vi "LDA_header.vi"() -> (0 "LDA Header string":string)   [LabVIEW 2010]
uses:
  Globals/Meas_global.vi
  Globals/LDA_meas_global_1.vi
  Globals/LDA_meas_global_2.vi
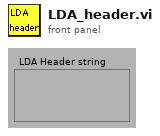
[diagram p1: front panel]
types:
  T1 = typedef "BSA_info_Cluster.ctl" = cluster{"GPIB Address":string, "No of Check Bytes":i32, "Extra Info":string, "COLOUR":u32, "Wavelength (nm)":dbl}
  T2 = cluster{"Arrival time clock":enum16{"External", "Internal"}, "Clock source":enum16{"Slave", "Master", "Private"}, "Coincidence":enum16{"Slave", "Master", "Private"}}
  T3 = cluster{"Dead time (s)":dbl, "Duty cycle (%)":dbl, "Data collection mode":enum16{"Burst", "Contiuous", "Dead time", "External"}}
  T4 = enum16{"Burst", "Contiuous", "Dead time", "External"}
  T5 = cluster{"Burst criterion":enum16{"Envelope", "Pedestal", "Env and ped"}, "Oversize reject level":enum16{"1 (disabled)", "2", "3", "4", "5", "6", "7", "8", "9"}, "Pedestal attenuation":enum16{"0", "6", "12", "18"}, "Record length":enum16{"8", "16", "32", "64"}, "Quality factor":i16}
  T6 = enum16{"1 (disabled)", "2", "3", "4", "5", "6", "7", "8", "9"}
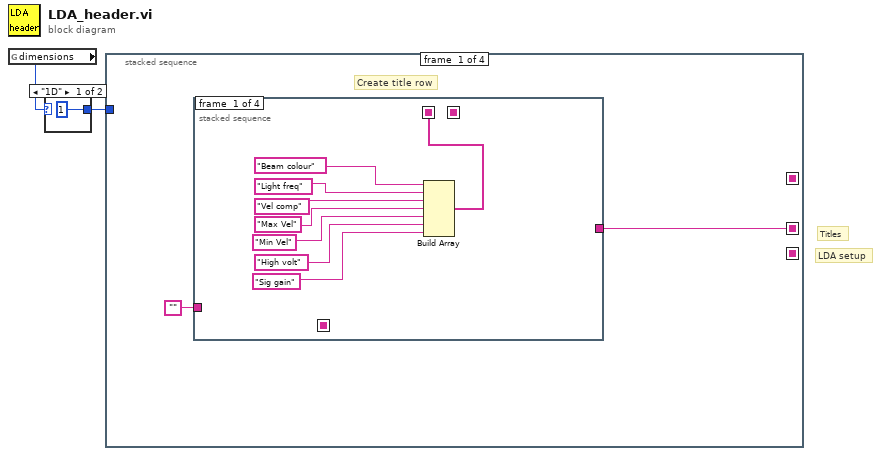
[diagram p0: block diagram]
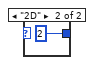
[diagram p2: hidden frame]
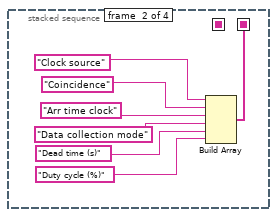
[diagram p3: hidden frame]
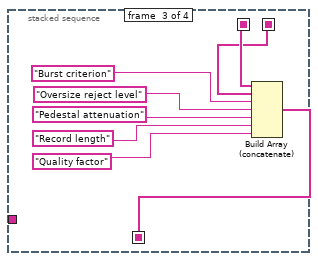
[diagram p4: hidden frame]
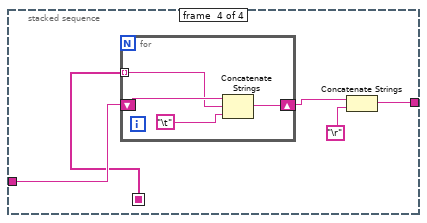
[diagram p5: hidden frame]
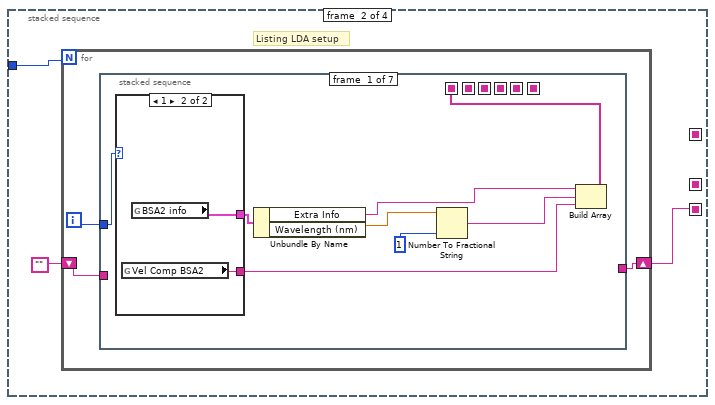
[diagram p6: hidden frame]
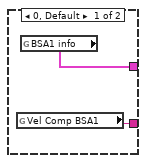
[diagram p7: hidden frame]
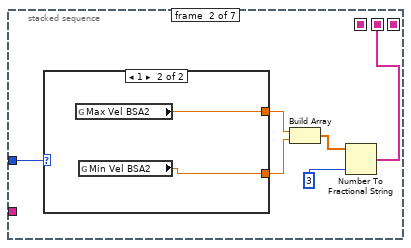
[diagram p8: hidden frame]
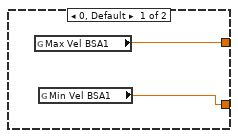
[diagram p9: hidden frame]
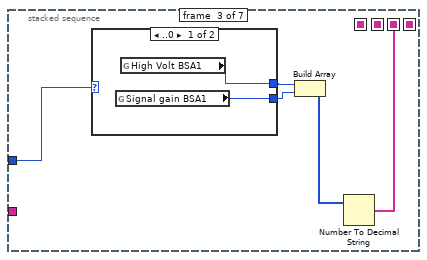
[diagram p10: hidden frame]
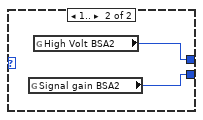
[diagram p11: hidden frame]
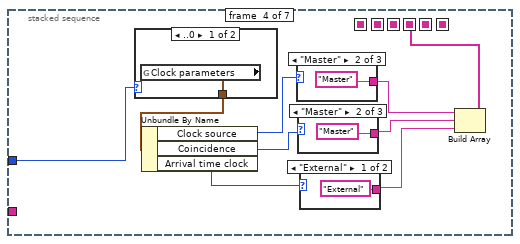
[diagram p12: hidden frame]
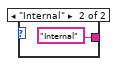
[diagram p13: hidden frame]
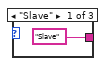
[diagram p14: hidden frame]
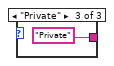
[diagram p15: hidden frame]
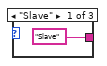
[diagram p16: hidden frame]
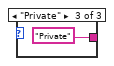
[diagram p17: hidden frame]
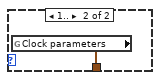
[diagram p18: hidden frame]
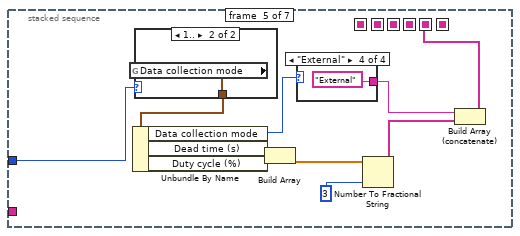
[diagram p19: hidden frame]
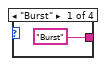
[diagram p20: hidden frame]
diagram:
  # "LDA setup"
  # "Titles"
  n1 = global read "Meas_global.vi" "dimensions"() -> (w2:enum16{"1D", "2D"})
  n2 = case shown="\"1D\"" w2 {
    tunnel: [1 2] -> w1
    frame "1D" {
    }
    frame "2D" {
    }
  }
  n3 = stacked-sequence {
    seq-local: [w6 _ _ _] -> [_ _ _ w174]
    seq-local: [_ w41 _ _] -> [_ _ _ w173]
    seq-local: [_ _ w164 _] -> [_ _ _ w176]
    tunnel: w1 -> [_ w39 _ _]
    frame #0 {
      # "Create title row"
      n4 = stacked-sequence {
        seq-local: [w7 _ _ _] -> [_ _ w24 _]
        seq-local: [_ w15 _ _] -> [_ _ w23 _]
        seq-local: [_ _ w22 _] -> [_ _ _ w33]
        tunnel: "" -> [_ _ _ w34]
        tunnel: [_ _ _ w31] -> w6
        frame #0 {
          n5 = Build Array("Beam colour", "Light freq", "Vel comp", "Max Vel", "Min Vel", "High volt", "Sig gain") -> (w7:string[])
        }
        frame #1 {
          n6 = Build Array("Clock source", "Coincidence", "Arr time clock", "Data collection mode", "Dead time (s)", "Duty cycle (%)") -> (w15:string[])
        }
        frame #2 {
          n7 = Build Array (concatenate)(w24, w23, "Burst criterion", "Oversize reject level", "Pedestal attenuation", "Record length", "Quality factor") -> (w22:string[])
        }
        frame #3 {
          n8 = for {
            shift-right: [w37] -> w32
            shift-left: w34 -> [w38]
            tunnel: w33 -> [w35] mode=indexing
            n9 = Concatenate Strings(w38, w35, "\t") -> (w37:string)
          }
          n10 = Concatenate Strings(w32, "\r") -> (w31:string)
        }
      }
    }
    frame #1 {
      # "Listing LDA setup"
      n11 = for {
        N: w39 -> [_]
        shift-right: [w42] -> w41
        shift-left: "" -> [w43]
        i -> [w44]
        n12 = stacked-sequence {
          seq-local: [_ w61 _ _ _ _ _] -> [_ _ _ _ _ _ w155]
          seq-local: [w48 _ _ _ _ _ _] -> [_ _ _ _ _ _ w156]
          seq-local: [_ _ w69 _ _ _ _] -> [_ _ _ _ _ _ w154]
          seq-local: [_ _ _ w76 _ _ _] -> [_ _ _ _ _ _ w153]
          seq-local: [_ _ _ _ w95 _ _] -> [_ _ _ _ _ _ w152]
          seq-local: [_ _ _ _ _ w111 _] -> [_ _ _ _ _ _ w151]
          tunnel: w44 -> [w52 w57 w71 w84 w104 w123 _]
          tunnel: w43 -> [_ _ _ _ _ _ w149]
          tunnel: [_ _ _ _ _ _ w148] -> w42
          frame #0 {
            n13 = case shown="1" w52 {
              tunnel: [w54 w56] -> w47
              tunnel: [w53 w55] -> w46
              frame 0, Default {
                n14 = global read "LDA_meas_global_1.vi" "Vel Comp BSA1"() -> (w53:string)
                n15 = global read "LDA_meas_global_1.vi" "BSA1 info"() -> (w54:T1)
              }
              frame 1 {
                n16 = global read "LDA_meas_global_2.vi" "Vel Comp BSA2"() -> (w55:string)
                n17 = global read "LDA_meas_global_2.vi" "BSA2 info"() -> (w56:T1)
              }
            }
            n18 = Unbundle By Name(w47) -> ("Extra Info"=w45:string, "Wavelength (nm)"=w50:dbl)
            n19 = Number To Fractional String(number=w50, precision (6)=1) -> (F-format string=w49:string)  [unwired: 2 out]
            n20 = Build Array(w45, w49, w46) -> (w48:string[])
          }
          frame #1 {
            n21 = case shown="1" w57 {
              tunnel: [w64 w66] -> w60
              tunnel: [w63 w65] -> w59
              frame 0, Default {
                n22 = global read "LDA_meas_global_1.vi" "Max Vel BSA1"() -> (w64:dbl)
                n23 = global read "LDA_meas_global_1.vi" "Min Vel BSA1"() -> (w63:dbl)
              }
              frame 1 {
                n24 = global read "LDA_meas_global_2.vi" "Max Vel BSA2"() -> (w66:dbl)
                n25 = global read "LDA_meas_global_2.vi" "Min Vel BSA2"() -> (w65:dbl)
              }
            }
            n26 = Build Array(w60, w59) -> (w58:dbl[])
            n27 = Number To Fractional String(number=w58, precision (6)=3) -> (F-format string=w61:string[])  [unwired: 2 out]
          }
          frame #2 {
            n28 = case shown="..0" w71 {
              tunnel: [w73 w75] -> w68
              tunnel: [w72 w74] -> w67
              frame ..0 {
                n29 = global read "LDA_meas_global_1.vi" "Signal gain BSA1"() -> (w72:i16)
                n30 = global read "LDA_meas_global_1.vi" "High Volt BSA1"() -> (w73:i16)
              }
              frame 1.. {
                n31 = global read "LDA_meas_global_2.vi" "Signal gain BSA2"() -> (w74:i16)
                n32 = global read "LDA_meas_global_2.vi" "High Volt BSA2"() -> (w75:i16)
              }
            }
            n33 = Build Array(w68, w67) -> (w70:i16[])
            n34 = Number To Decimal String(number=w70) -> (decimal integer string=w69:string[])  [unwired: 1 out]
          }
          frame #3 {
            n35 = case shown="..0" w84 {
              tunnel: [w93 w94] -> w83
              frame ..0 {
                n36 = global read "LDA_meas_global_1.vi" "Clock parameters"() -> (w93:T2)
              }
              frame 1.. {
                n37 = global read "LDA_meas_global_2.vi" "Clock parameters"() -> (w94:T2)
              }
            }
            n38 = Unbundle By Name(w83) -> ("Clock source"=w81:enum16{"Slave", "Master", "Private"}, "Coincidence"=w82:enum16{"Slave", "Master", "Private"}, "Arrival time clock"=w78:enum16{"External", "Internal"})
            n39 = case shown="\"Master\"" w81 {
              tunnel: ["Slave" "Master" "Private"] -> w80
              frame "Slave" {
              }
              frame "Master" {
              }
              frame "Private" {
              }
            }
            n40 = case shown="\"Master\"" w82 {
              tunnel: ["Slave" "Master" "Private"] -> w79
              frame "Slave" {
              }
              frame "Master" {
              }
              frame "Private" {
              }
            }
            n41 = case shown="\"External\"" w78 {
              tunnel: ["External" "Internal"] -> w77
              frame "External" {
              }
              frame "Internal" {
              }
            }
            n42 = Build Array(w80, w79, w77) -> (w76:string[])
          }
          frame #4 {
            n43 = case shown="1.." w104 {
              tunnel: [w109 w110] -> w103
              frame ..0 {
                n44 = global read "LDA_meas_global_1.vi" "Data collection mode"() -> (w109:T3)
              }
              frame 1.. {
                n45 = global read "LDA_meas_global_2.vi" "Data collection mode"() -> (w110:T3)
              }
            }
            n46 = Unbundle By Name(w103) -> ("Data collection mode"=w102:T4, "Dead time (s)"=w98:dbl, "Duty cycle (%)"=w97:dbl)
            n47 = Build Array(w98, w97) -> (w99:dbl[])
            n48 = case shown="\"External\"" w102 {
              tunnel: ["Burst" "Continuous" "Dead time" "External"] -> w101
              frame "Burst" {
              }
              frame "Contiuous" {
              }
              frame "Dead time" {
              }
              frame "External" {
              }
            }
            n49 = Number To Fractional String(number=w99, precision (6)=3) -> (F-format string=w96:string[])  [unwired: 2 out]
            n50 = Build Array (concatenate)(w101, w96) -> (w95:string[])
          }
          frame #5 {
            n51 = case shown="1.." w123 {
              tunnel: [w144 w145] -> w122
              frame ..0 {
                n52 = global read "LDA_meas_global_1.vi" "Analysis parameters"() -> (w144:T5)
              }
              frame 1.. {
                n53 = global read "LDA_meas_global_2.vi" "Analysis parameters"() -> (w145:T5)
              }
            }
            n54 = Unbundle By Name(w122) -> ("Burst criterion"=w120:enum16{"Envelope", "Pedestal", "Env and ped"}, "Oversize reject level"=w121:T6, "Pedestal attenuation"=w117:enum16{"0", "6", "12", "18"}, "Record length"=w115:enum16{"8", "16", "32", "64"}, "Quality factor"=w114:i16)
            n55 = case shown="\"Envelope\"" w120 {
              tunnel: ["Envelope" "Pedestal" "Env and ped"] -> w119
              frame "Envelope" {
              }
              frame "Pedestal" {
              }
              frame "Env and ped" {
              }
            }
            n56 = case shown="\"1 (disabled)\"" w121 {
              tunnel: ["1 (disabled)" "2" "3" "4" "5" "6" "7" "8" "9"] -> w118
              frame "1 (disabled)" {
              }
              frame "2" {
              }
              frame "3" {
              }
              frame "4" {
              }
              frame "5" {
              }
              frame "6" {
              }
              frame "7" {
              }
              frame "8" {
              }
              frame "9" {
              }
            }
            n57 = case shown="\"0\"" w117 {
              tunnel: ["0" "6" "12" "18"] -> w116
              frame "0" {
              }
              frame "6" {
              }
              frame "12" {
              }
              frame "18" {
              }
            }
            n58 = Number To Decimal String(number=w114) -> (decimal integer string=w113:string)  [unwired: 1 out]
            n59 = case shown="\"64\"" w115 {
              tunnel: ["8" "16" "32" "64"] -> w112
              frame "8" {
              }
              frame "16" {
              }
              frame "32" {
              }
              frame "64" {
              }
            }
            n60 = Build Array(w119, w118, w116, w112, w113) -> (w111:string[])
          }
          frame #6 {
            n61 = Build Array (concatenate)(w156, w155, w154, w153, w152, w151) -> (w150:string[])
            n62 = for {
              shift-right: [w159] -> w146
              shift-left: w149 -> [w160]
              tunnel: w150 -> [w157] mode=indexing
              n63 = Concatenate Strings(w160, w157, "\t") -> (w159:string)
            }
            n64 = Concatenate Strings(w146, "\r") -> (w148:string)
          }
        }
      }
    }
    frame #2 {
      n65 = global read "Meas_global.vi" "Analogue data"() -> (w165:enum16{"No Analogue data", "Take Analogue data"})
      n66 = case shown="\"Take Analogue data\"" w165 {
        tunnel: ["" w169] -> w162
        frame "No Analogue data" {
        }
        frame "Take Analogue data" {
          n67 = global read "Meas_global.vi" "Synchronise with LDA"() -> (w170:bool)
          n68 = case shown="True" w170 {
            tunnel: ["Analogue data is not synchronised with the LDA" "Analogue data is synchronised with the LDA"] -> w168
            frame False {
            }
            frame True {
            }
          }
          n69 = Concatenate Strings(w168, "\r") -> (w169:string)
        }
      }
      n70 = global read "LDA_meas_global_1.vi" "Probe Configuration"() -> (w161:string)
      n71 = Concatenate Strings(w161, "\r", w162) -> (w164:string)
    }
    frame #3 {
      n72 = Concatenate Strings(w176, w174, w173) -> (→"LDA Header string":string)
    }
  }
